vi "testError.vi"() -> (0 "error out":errorcluster)   [LabVIEW 2019, in "AssertionTest.lvlib" / "AssertFalse.lvlib"]
uses:
  AssertFalse.lvlib
  <vilib>/Utility/error.llb/Error Cluster From Error Code.vi
  <vilib>/ErrorRing/Error Ring.xnode
  AssertionTest.lvlib
  Assertion/Assertion.lvlib
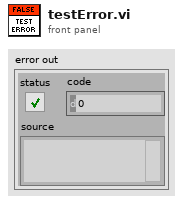
[diagram p1: front panel]
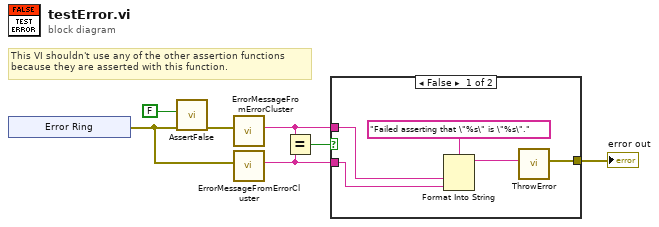
[diagram p0: block diagram]
diagram:
  # "This VI shouldn't use any of the other assertion functions\nbecause they are asserted with this function."
  n1 = xnode "Error Ring"() -> ("error out"=w5:errorcluster)
  n2 = call "AssertFalse.vi"("error in (no error)"=w5, "Condition"=FALSE) -> ("error out"=w6:errorcluster)  [unwired: 9 in]
  n3 = call "ErrorMessageFromErrorCluster.vi"("Error"=w6) -> ("Error Message"=w3:string)  [unwired: 10 in]
  n4 = call "ErrorMessageFromErrorCluster.vi"("Error"=w5) -> ("Error Message"=w2:string)  [unwired: 10 in]
  n5 = Equal?(x=w3, y=w2) -> (x = y?=w4:bool)
  n6 = case shown="False" w4 {
    tunnel: w3 -> [w11 _]
    tunnel: w2 -> [w10 _]
    tunnel: [w8 _] -> w1
    frame False {
      n7 = Format Into String(format string="Failed asserting that \"%s\" is \"%s\".", w11, w10) -> (resulting string=w9:string)  [unwired: 2 in, 1 out]
      n8 = call "ThrowError.vi"("Error Message"=w9) -> ("error out"=w8:errorcluster)  [unwired: 10 in]
    }
    frame True {
    }
  }
  "error out" <- w1
